vi "_FPGA Get System Status.vi"(6 "Server State":string) -> (2 "Status":string)   [LabVIEW 2015]
uses:
  Type/_RT Instrument State.ctl
  _RT Global.vi
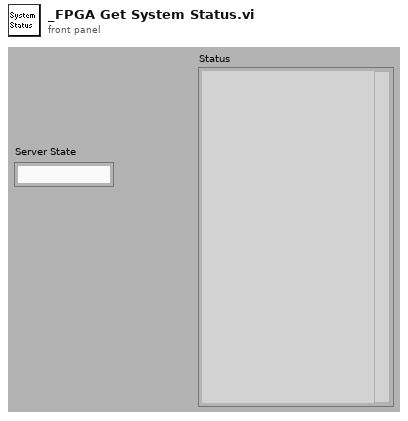
[diagram p1: front panel]
types:
  T1 = typedef "_RT Instrument State.ctl" = enum16{"Initializing", "Mass Spectrometer is Off", "Starting Up", "Turning Power Off", "Going to Standby", "Roughing Pump Ready", "Turning Turbo Off", "Turbo Startup", "Turbopump Ready", "Checking Vacuum", "Going to Ready", "Ready", "Running", "Source Standby", "Lost Communication", "Shutting Down", "Fault", "24V Standby", "Go to 24V Standby", "Turbopump Ready-Waiting"}
  T2 = typedef "_RT Startup Options.ctl" = cluster{"Door":bool, "Curtain":bool, "Pressure":bool, "Turbo":bool, "SysPoll":bool, "GasFlag":bool}
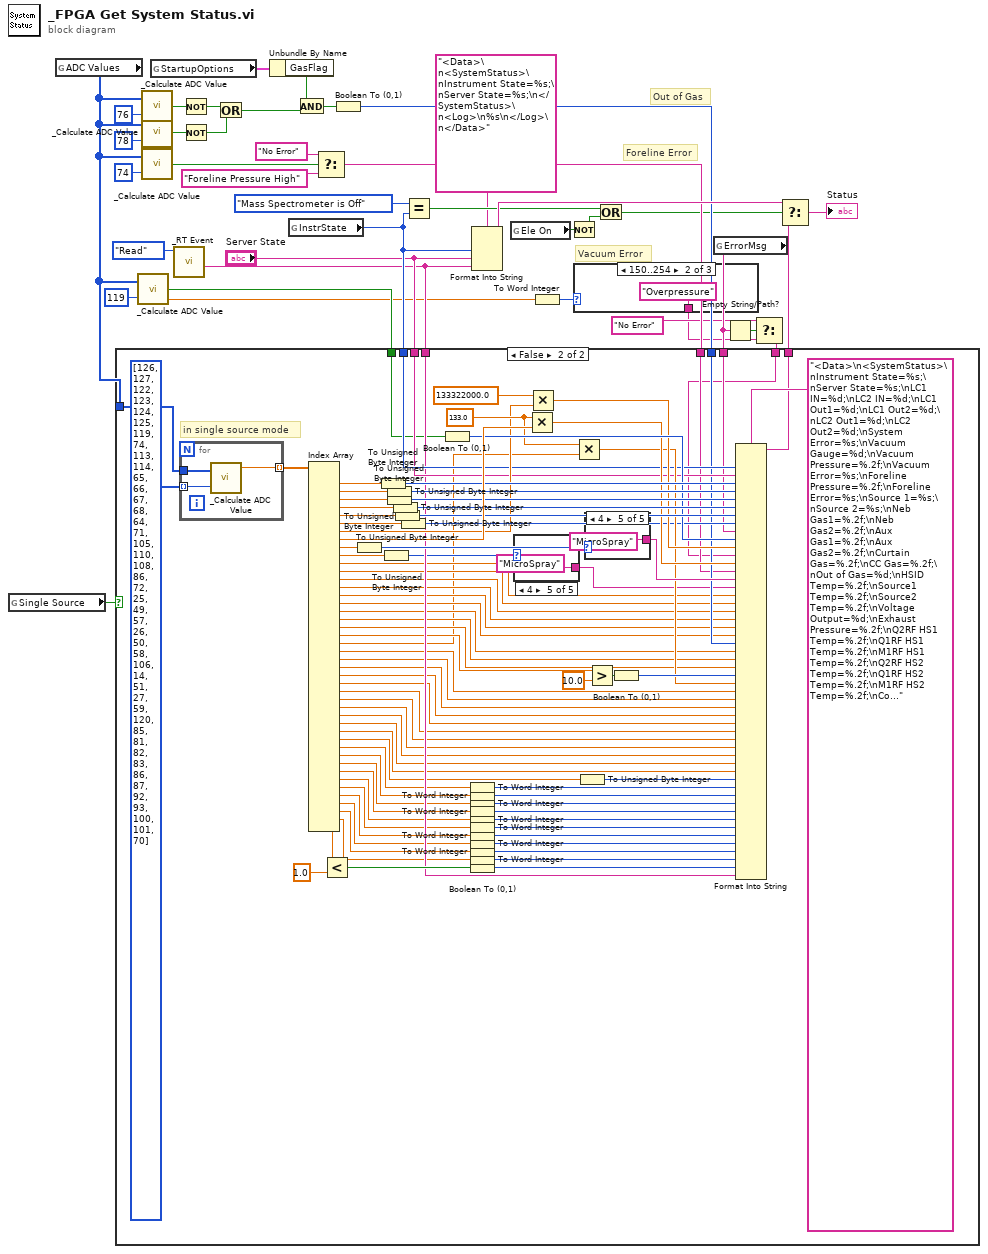
[diagram p0: block diagram]
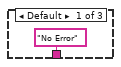
[diagram p2: hidden frame]
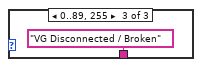
[diagram p3: hidden frame]
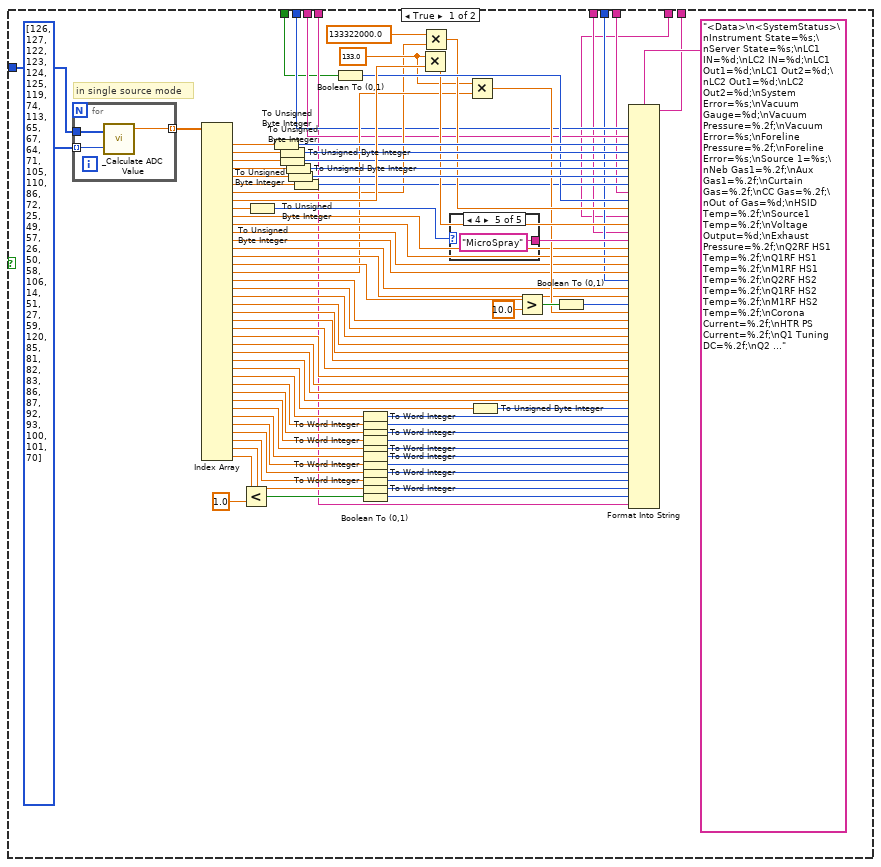
[diagram p4: hidden frame]
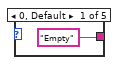
[diagram p5: hidden frame]
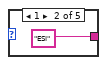
[diagram p6: hidden frame]
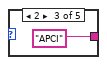
[diagram p7: hidden frame]
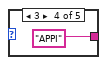
[diagram p8: hidden frame]
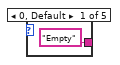
[diagram p9: hidden frame]
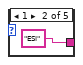
[diagram p10: hidden frame]
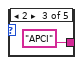
[diagram p11: hidden frame]
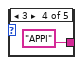
[diagram p12: hidden frame]
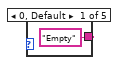
[diagram p13: hidden frame]
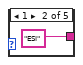
[diagram p14: hidden frame]
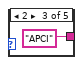
[diagram p15: hidden frame]
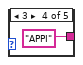
[diagram p16: hidden frame]
diagram:
  # "Vacuum Error"
  # "Foreline Error"
  # "Out of Gas"
  n1 = global read "_RT Global.vi" "Single Source"() -> (w40:bool)
  n2 = global read "_RT Global.vi" "ADC Values"() -> (w10:i32[])
  n3 = call "_Calculate ADC Value.vi"("ADC Values"=w10, "ADC Channel (64)"=u8 119) -> ("In Range?"=w28:bool, "Raw Reading"=w26:sgl)  [unwired: 1 out]
  n4 = call "_Calculate ADC Value.vi"("ADC Values"=w10, "ADC Channel (64)"=u8 76) -> ("In Range?"=w20:bool)  [unwired: 2 out]
  n5 = call "_Calculate ADC Value.vi"("ADC Values"=w10, "ADC Channel (64)"=u8 78) -> ("In Range?"=w21:bool)  [unwired: 2 out]
  n6 = call "_Calculate ADC Value.vi"("ADC Values"=w10, "ADC Channel (64)"=u8 74) -> ("In Range?"=w12:bool)  [unwired: 2 out]
  n7 = global read "_RT Global.vi" "StartupOptions"() -> (w24:T2)
  n8 = call "_RT Event.vi"("Action (Write)"=enum16{"Write", "Read"}."Read") -> ("Log"=w30:string)  [unwired: 2 in, 4 out]
  n9 = Not(x=w20) -> (.not. x?=w22:bool)
  n10 = Not(x=w21) -> (.not. x?=w23:bool)
  n11 = Or(x=w22, y=w23) -> (x .or. y?=w16:bool)
  n12 = Unbundle By Name(w24) -> ("GasFlag"=w17:bool)
  n13 = global read "_RT Global.vi" "InstrState"() -> (w34:T1)
  n14 = And(x=w17, y=w16) -> (x .and. y?=w25:bool)
  n15 = Select(t="No Error" ("input 12"), s=w12, f="Foreline Pressure High" ("input 12")) -> (s? t:f=w9:string)
  n16 = Boolean To (0,1)(Boolean=w25) -> (0, 1=w15:i16)
  n17 = Equal?(x=_RT_Instrument_State."Mass Spectrometer is Off", y=w34) -> (x = y?=w37:bool)
  n18 = Format Into String(format string="<Data>\n<SystemStatus>\nInstrument State=%s;\nServer State=%s;\n</SystemStatus>\n<Log>\n%s\n</Log>\n</Data>", w34, "Server State", w30) -> (resulting string=w38:string)  [unwired: 2 in, 1 out]
  n19 = global read "_RT Global.vi" "Ele On"() -> (w6:bool)
  n20 = To Word Integer(number=w26) -> (16bit integer=w27:i16)
  n21 = Not(x=w6) -> (.not. x?=w7:bool)
  n22 = case shown="150..254" w27 {
    tunnel: ["No Error" "Overpressure" "VG Disconnected / Broken"] -> w2
    frame Default {
    }
    frame 150..254 {
    }
    frame 0..89, 255 {
    }
  }
  n23 = Or(x=w37, y=w7) -> (x .or. y?=w8:bool)
  n24 = global read "_RT Global.vi" "ErrorMsg"() -> (w5:string)
  n25 = Empty String/Path?(string/path=w5) -> (empty?=w4:bool)
  n26 = Select(t="No Error", s=w4, f=w2) -> (s? t:f=w1:string)
  n27 = case shown="False" w40 {
    tunnel: w34 -> [w53 w182]
    tunnel: "Server State" -> [w52 w181]
    tunnel: w30 -> [w51 w180]
    tunnel: [w50 w179] -> w33
    tunnel: w5 -> [w49 w178]
    tunnel: w10 -> [w48 w177]
    tunnel: w28 -> [w47 w176]
    tunnel: w15 -> [w46 w175]
    tunnel: w9 -> [w45 w174]
    tunnel: w1 -> [w44 w136]
    frame True {
      w89 = sgl 133.0 ("y")
      # "in single source mode"
      n28 = for {
        tunnel: w48 -> [w135]
        tunnel: u8[] [126, 127, 122, 123, 124, 125, 119, 74, 113, 65, 67, 64, 71, 105, 110, 86, 72, 25, 49, 57, 26, 50, 58, 106, 14, 51, 27, 59, 120, 85, 81, 82, 83, 86, 87, 92, 93, 100, 101, 70] -> [w134] mode=indexing
        tunnel: [w133] -> w126 mode=indexing
        n29 = call "_Calculate ADC Value.vi"("ADC Values"=w135, "ADC Channel (64)"=w134) -> ("User Value"=w133:sgl)  [unwired: 2 out]
      }
      n30 = Index Array(array=w126) -> (element #1=w125:sgl, element #2=w124:sgl, element #3=w123:sgl, element #4=w122:sgl, element #5=w121:sgl, element #6=w120:sgl, element #7=w54:sgl, element #8=w119:sgl, element #9=w118:sgl, element #10=w85:sgl, element #11=w84:sgl, element #12=w83:sgl, element #13=w82:sgl, element #14=w81:sgl, element #15=w80:sgl, element #16=w79:sgl, element #17=w78:sgl, element #18=w77:sgl, element #19=w76:sgl, element #20=w75:sgl, element #21=w74:sgl, element #22=w73:sgl, element #23=w72:sgl, element #24=w71:sgl, element #25=w70:sgl, element #26=w69:sgl, element #27=w68:sgl, element #28=w67:sgl, element #29=w66:sgl, element #30=w65:sgl, element #31=w64:sgl, element #32=w63:sgl, element #33=w62:sgl, element #34=w61:sgl, element #35=w60:sgl, element #36=w59:sgl, element #37=w58:sgl, element #38=w57:sgl, element #39=w56:sgl, element #40=w55:sgl)  [unwired: 40 in]
      n31 = Less?(x=w55, y=sgl 1.0) -> (x < y?=w87:bool)
      n32 = To Unsigned Byte Integer(number=w118) -> (unsigned 8bit integer=w117:u8)
      n33 = To Unsigned Byte Integer(number=w125) -> (unsigned 8bit integer=w115:u8)
      n34 = To Unsigned Byte Integer(number=w124) -> (unsigned 8bit integer=w114:u8)
      n35 = To Unsigned Byte Integer(number=w123) -> (unsigned 8bit integer=w113:u8)
      n36 = To Unsigned Byte Integer(number=w122) -> (unsigned 8bit integer=w112:u8)
      n37 = To Unsigned Byte Integer(number=w121) -> (unsigned 8bit integer=w111:u8)
      n38 = To Unsigned Byte Integer(number=w120) -> (unsigned 8bit integer=w90:u8)
      n39 = Boolean To (0,1)(Boolean=w47) -> (0, 1=w110:i16)
      n40 = To Word Integer(number=w65) -> (16bit integer=w100:i16)
      n41 = To Word Integer(number=w64) -> (16bit integer=w98:i16)
      n42 = To Word Integer(number=w63) -> (16bit integer=w97:i16)
      n43 = To Word Integer(number=w62) -> (16bit integer=w96:i16)
      n44 = To Word Integer(number=w61) -> (16bit integer=w95:i16)
      n45 = To Word Integer(number=w60) -> (16bit integer=w94:i16)
      n46 = To Word Integer(number=w59) -> (16bit integer=w93:i16)
      n47 = To Word Integer(number=w58) -> (16bit integer=w92:i16)
      n48 = To Word Integer(number=w57) -> (16bit integer=w91:i16)
      n49 = To Word Integer(number=w56) -> (16bit integer=w99:i16)
      n50 = Boolean To (0,1)(Boolean=w87) -> (0, 1=w86:i16)
      n51 = Multiply(x=w89, y=w119) -> (x*y=w108:sgl)
      n52 = Multiply(x=sgl 133322000.0 ("y"), y=w54) -> (x*y=w109:sgl)
      n53 = case shown="4" w117 {
        tunnel: ["Empty" "ESI" "APCI" "APPI" "MicroSpray"] -> w107
        frame 0, Default {
        }
        frame 1 {
        }
        frame 2 {
        }
        frame 3 {
        }
        frame 4 {
        }
      }
      n54 = Multiply(x=w89, y=w78) -> (x*y=w102:sgl)
      n55 = To Unsigned Byte Integer(number=w66) -> (unsigned 8bit integer=w101:u8)
      n56 = Greater?(x=w79, y=sgl 10.0) -> (0:w105:bool)
      n57 = Boolean To (0,1)(Boolean=w105) -> (0, 1=w104:i16)
      n58 = Format Into String(format string="<Data>\n<SystemStatus>\nInstrument State=%s;\nServer State=%s;\nLC1 IN=%d;\nLC2 IN=%d;\nLC1 Out1=%d;\nLC1 Out2=%d;\nLC2 Out1=%d;\nLC2 Out2=%d;\nSystem Error=%s;\nVacuum Gauge=%d;\nVacuum Pressure=%.2f;\nVacuum Error=%s;\nForeline Pressure=%.2f;\nForeline Error=%s;\nSource 1=%s;\nNeb Gas1=%.2f;\nAux Gas1=%.2f;\nCurtain Gas=%.2f;\nCC Gas=%.2f;\nOut of Gas=%d;\nHSID Temp=%.2f;\nSource1 Temp=%.2f;\nVoltage Output=%d;\nExhaust Pressure=%.2f;\nQ2RF HS1 Temp=%.2f;\nQ1RF HS1 Temp=%.2f;\nM1RF HS1 Temp=%.2f;\nQ2RF HS2 Temp=%.2f;\nQ1RF HS2 Temp=%.2f;\nM1RF HS2 Temp=%.2f;\nCorona Current=%.2f;\nHTR PS Current=%.2f;\nQ1 Tuning DC=%.2f;\nQ2 Tuning DC=%.2f;\nM1RF Tuning DC=%.2f;\nDoor Interlock=%d;\n24V=%d;\n28V=%d;\n-28V=%d;\n60V=%d;\n15V=%d;\n-15V=%d;\nLens Board 2 +5V=%d;\nLens Board 2 -5V=%d;\nLens Board 1 +5V=%d;\nLens Board 1 -5V=%d;\nSource Exhaust Valve=%d;\n</SystemStatus>\n<Log>\n%s\n</Log>\n</Data>", w53, w52, w115, w114, w113, w112, w111, w90, w49, w110, w109, w44, w108, w45, w107, w85, w84, w83, w82, w46, w81, w80, w104, w102, w77, w76, w75, w74, w73, w72, w71, w70, w69, w68, w67, w101, w100, w98, w97, w96, w95, w94, w93, w92, w91, w99, w86, w51) -> (resulting string=w50:string)  [unwired: 2 in, 1 out]
    }
    frame False {
      w187 = sgl 133.0 ("y")
      # "in single source mode"
      n59 = for {
        tunnel: w177 -> [w238]
        tunnel: u8[] [126, 127, 122, 123, 124, 125, 119, 74, 113, 114, 65, 66, 67, 68, 64, 71, 105, 110, 108, 86, 72, 25, 49, 57, 26, 50, 58, 106, 14, 51, 27, 59, 120, 85, 81, 82, 83, 86, 87, 92, 93, 100, 101, 70] -> [w237] mode=indexing
        tunnel: [w236] -> w224 mode=indexing
        n60 = call "_Calculate ADC Value.vi"("ADC Values"=w238, "ADC Channel (64)"=w237) -> ("User Value"=w236:sgl)  [unwired: 2 out]
      }
      n61 = Index Array(array=w224) -> (element #1=w223:sgl, element #2=w222:sgl, element #3=w221:sgl, element #4=w220:sgl, element #5=w219:sgl, element #6=w218:sgl, element #7=w183:sgl, element #8=w217:sgl, element #9=w216:sgl, element #10=w172:sgl, element #11=w173:sgl, element #12=w168:sgl, element #13=w167:sgl, element #14=w166:sgl, element #15=w165:sgl, element #16=w164:sgl, element #17=w163:sgl, element #18=w162:sgl, element #19=w161:sgl, element #20=w160:sgl, element #21=w159:sgl, element #22=w158:sgl, element #23=w157:sgl, element #24=w156:sgl, element #25=w155:sgl, element #26=w154:sgl, element #27=w153:sgl, element #28=w152:sgl, element #29=w151:sgl, element #30=w150:sgl, element #31=w149:sgl, element #32=w148:sgl, element #33=w147:sgl, element #34=w146:sgl, element #35=w145:sgl, element #36=w144:sgl, element #37=w143:sgl, element #38=w142:sgl, element #39=w141:sgl, element #40=w140:sgl, element #41=w139:sgl, element #42=w138:sgl, element #43=w137:sgl, element #44=w169:sgl)  [unwired: 44 in]
      n62 = Less?(x=w169, y=sgl 1.0) -> (x < y?=w185:bool)
      n63 = To Unsigned Byte Integer(number=w216) -> (unsigned 8bit integer=w215:u8)
      n64 = To Unsigned Byte Integer(number=w223) -> (unsigned 8bit integer=w213:u8)
      n65 = To Unsigned Byte Integer(number=w172) -> (unsigned 8bit integer=w170:u8)
      n66 = To Unsigned Byte Integer(number=w222) -> (unsigned 8bit integer=w212:u8)
      n67 = To Unsigned Byte Integer(number=w221) -> (unsigned 8bit integer=w211:u8)
      n68 = To Unsigned Byte Integer(number=w220) -> (unsigned 8bit integer=w210:u8)
      n69 = To Unsigned Byte Integer(number=w219) -> (unsigned 8bit integer=w209:u8)
      n70 = To Unsigned Byte Integer(number=w218) -> (unsigned 8bit integer=w188:u8)
      n71 = Boolean To (0,1)(Boolean=w176) -> (0, 1=w208:i16)
      n72 = To Word Integer(number=w146) -> (16bit integer=w198:i16)
      n73 = To Word Integer(number=w145) -> (16bit integer=w196:i16)
      n74 = To Word Integer(number=w144) -> (16bit integer=w195:i16)
      n75 = To Word Integer(number=w143) -> (16bit integer=w194:i16)
      n76 = To Word Integer(number=w142) -> (16bit integer=w193:i16)
      n77 = To Word Integer(number=w141) -> (16bit integer=w192:i16)
      n78 = To Word Integer(number=w140) -> (16bit integer=w191:i16)
      n79 = To Word Integer(number=w139) -> (16bit integer=w190:i16)
      n80 = To Word Integer(number=w138) -> (16bit integer=w189:i16)
      n81 = To Word Integer(number=w137) -> (16bit integer=w197:i16)
      n82 = Boolean To (0,1)(Boolean=w185) -> (0, 1=w184:i16)
      n83 = case shown="4" w170 {
        tunnel: ["Empty" "ESI" "APCI" "APPI" "MicroSpray"] -> w171
        frame 0, Default {
        }
        frame 1 {
        }
        frame 2 {
        }
        frame 3 {
        }
        frame 4 {
        }
      }
      n84 = Multiply(x=w187, y=w217) -> (x*y=w206:sgl)
      n85 = Multiply(x=sgl 133322000.0 ("y"), y=w183) -> (x*y=w207:sgl)
      n86 = Multiply(x=w187, y=w159) -> (x*y=w200:sgl)
      n87 = To Unsigned Byte Integer(number=w147) -> (unsigned 8bit integer=w199:u8)
      n88 = case shown="4" w215 {
        tunnel: ["Empty" "ESI" "APCI" "APPI" "MicroSpray"] -> w205
        frame 0, Default {
        }
        frame 1 {
        }
        frame 2 {
        }
        frame 3 {
        }
        frame 4 {
        }
      }
      n89 = Greater?(x=w160, y=sgl 10.0) -> (0:w203:bool)
      n90 = Boolean To (0,1)(Boolean=w203) -> (0, 1=w202:i16)
      n91 = Format Into String(format string="<Data>\n<SystemStatus>\nInstrument State=%s;\nServer State=%s;\nLC1 IN=%d;\nLC2 IN=%d;\nLC1 Out1=%d;\nLC1 Out2=%d;\nLC2 Out1=%d;\nLC2 Out2=%d;\nSystem Error=%s;\nVacuum Gauge=%d;\nVacuum Pressure=%.2f;\nVacuum Error=%s;\nForeline Pressure=%.2f;\nForeline Error=%s;\nSource 1=%s;\nSource 2=%s;\nNeb Gas1=%.2f;\nNeb Gas2=%.2f;\nAux Gas1=%.2f;\nAux Gas2=%.2f;\nCurtain Gas=%.2f;\nCC Gas=%.2f;\nOut of Gas=%d;\nHSID Temp=%.2f;\nSource1 Temp=%.2f;\nSource2 Temp=%.2f;\nVoltage Output=%d;\nExhaust Pressure=%.2f;\nQ2RF HS1 Temp=%.2f;\nQ1RF HS1 Temp=%.2f;\nM1RF HS1 Temp=%.2f;\nQ2RF HS2 Temp=%.2f;\nQ1RF HS2 Temp=%.2f;\nM1RF HS2 Temp=%.2f;\nCorona Current=%.2f;\nHTR PS Current=%.2f;\nQ1 Tuning DC=%.2f;\nQ2 Tuning DC=%.2f;\nM1RF Tuning DC=%.2f;\nDoor Interlock=%d;\n24V=%d;\n28V=%d;\n-28V=%d;\n60V=%d;\n15V=%d;\n-15V=%d;\nLens Board 2 +5V=%d;\nLens Board 2 -5V=%d;\nLens Board 1 +5V=%d;\nLens Board 1 -5V=%d;\nSource Exhaust Valve=%d;\n</SystemStatus>\n<Log>\n%s\n</Log>\n</Data>", w182, w181, w213, w212, w211, w210, w209, w188, w178, w208, w207, w136, w206, w174, w205, w171, w173, w168, w167, w166, w165, w164, w175, w163, w162, w161, w202, w200, w158, w157, w156, w155, w154, w153, w152, w151, w150, w149, w148, w199, w198, w196, w195, w194, w193, w192, w191, w190, w189, w197, w184, w180) -> (resulting string=w179:string)  [unwired: 2 in, 1 out]
    }
  }
  n92 = Select(t=w38, s=w8, f=w33) -> (s? t:f=→"Status":string)
